vi "test_tcp.vi"() -> ()   [LabVIEW 2017]
panel:
  out "웨이브폼 차트":u32(graph)
  out "x-y":u32
  in  "정지":bool
  out "숫자":i32
  out "read_data":string
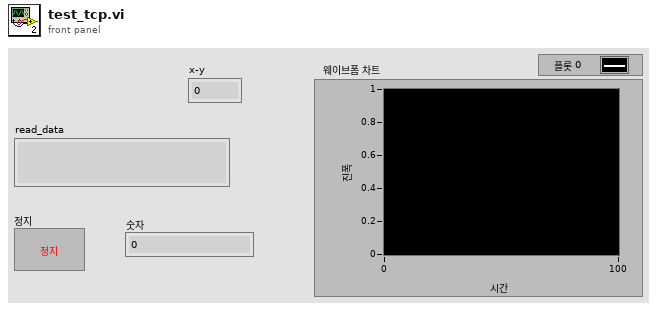
[diagram p1: front panel]
types:
  T1 = enum16{"Standard", "Buffered", "CRLF", "Immediate"}
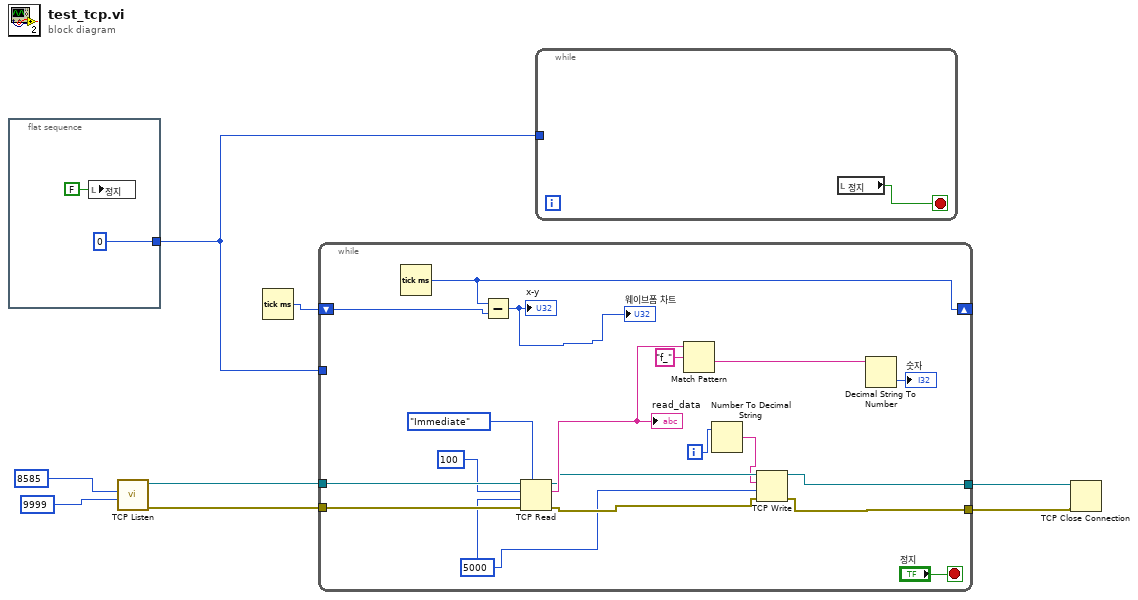
[diagram p0: block diagram]
diagram:
  n1 = flat-sequence {
    tunnel: [0] -> w8
    frame #0 {
      n2 = local write "정지"(FALSE ("정지")) -> ()
    }
  }
  n3 = call <vilib>:"TCP Listen.vi"("timeout ms (wait forever: -1)"=9999, "port"=u16 8585) -> ("error out"=w5:errorcluster, "connection ID"=w4:refnum<k5>)  [unwired: 5 in, 3 out]
  n4 = Tick Count (ms)() -> (millisecond timer value=w1:u32)
  n5 = while {
    tunnel: w5 -> [w24]
    tunnel: [w21] -> w3
    tunnel: w8 -> [_]
    tunnel: w4 -> [w25]
    tunnel: [w18] -> w2
    shift-right: [w14] -> _
    shift-left: w1 -> [w13]
    i -> [w16]
    stop <- "정지" stop-if-true
    w12 = 5000 ("타임아웃 ms (25000)")
    n6 = Tick Count (ms)() -> (millisecond timer value=w14:u32)
    n7 = Subtract(x=w14, y=w13) -> (x-y=→"x-y" →"웨이브폼 차트":u32)
    n8 = TCP Read(connection ID=w25, bytes to read=100 ("읽을 바이트"), error in (no error)=w24, 7:T1."Immediate" ("모드(standard)"), 9:w12) -> (connection ID out=w19:refnum<k5>, data out=w22:string, error out=w20:errorcluster)
    "read_data" <- w22
    n9 = Match Pattern(string=w22, regular expression="f_" ("정규식")) -> (after substring=w28:string)  [unwired: 1 in, 3 out]
    n10 = Number To Decimal String(number=w16) -> (decimal integer string=w15:string)  [unwired: 1 in]
    n11 = TCP Write(connection ID=w19, data in=w15, error in (no error)=w20, 9:w12) -> (connection ID out=w18:refnum<k5>, error out=w21:errorcluster)  [unwired: 1 out]
    n12 = Decimal String To Number(string=w28) -> (number=→"숫자":i32)  [unwired: 2 in, 1 out]
  }
  n13 = while {
    tunnel: w8 -> [_]
    stop <- w30 stop-if-true
    n14 = local read "정지"() -> (w30:bool)
  }
  n15 = TCP Close Connection(connection ID=w2, error in (no error)=w3) -> ()  [unwired: 3 out]
